vi "Set_OnlineData.vi"(8 "error in (no error)":errorcluster, 10 "Data_IN":T1={"Online"=TRUE, "Info"="", "OnlineData_State"=0} {"OnlineData_State" items=["Idle", "Manually", "Automatic"]}, 11 "MonSys_Server_Actor in":refnum<class "MonSys_Server_Actor.lvclass">) -> (0 "error out":errorcluster, 3 "MonSys_Server_Actor out":refnum<class "MonSys_Server_Actor.lvclass">)   [LabVIEW 2018, in "MonSys_Server_Actor.lvlib" / "MonSys_Server_Actor.lvclass"]
doc: "Replace SystemState DVR Data"
uses:
  MonSys_Server_Actor.lvclass
  _MonSys_LIB/OnlineData.ctl
  _MonSys_LIB/OnlineData_State.ctl
  MonSys_Server_Actor.lvclass/MonSys_Server_Actor.ctl
  _MonSys_LIB/_MonSys_LIB.lvlib
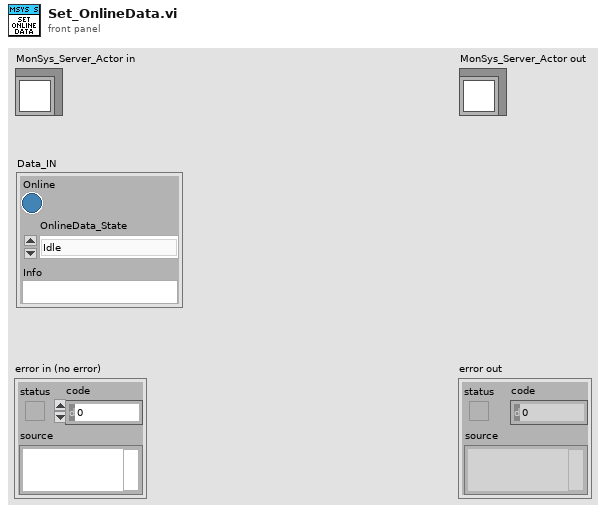
[diagram p1: front panel]
types:
  T1 = typedef "_MonSys_LIB.lvlib/OnlineData.ctl" = cluster{"Online":bool, "Info":string, "OnlineData_State":T2}
  T2 = typedef "_MonSys_LIB.lvlib/OnlineData_State.ctl" = u16
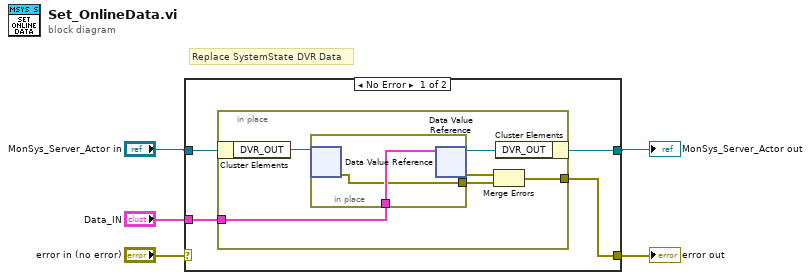
[diagram p0: block diagram]
diagram:
  # "Replace SystemState DVR Data"
  n1 = case shown="No Error" "error in (no error)" {
    selector: "error in (no error)" -> [_ w19]
    tunnel: [w7 w19] -> w3
    tunnel: [w6 w18] -> w2
    tunnel: "MonSys_Server_Actor in" -> [w9 w18]
    tunnel: "Data_IN" -> [w8 _]
    frame No Error {
      n2 = in-place {
        in-place-border: w8 -> [w14]
        in-place-border: [w11] -> w7
        n3 = in-place-cluster #1(w9) -> ("DVR_OUT"=w15:refnum<data-value>)
        n4 = in-place {
          in-place-border: w14 -> [w17]
          in-place-border: [w16] -> w13
          n5 = in-place-dvr #2(w15) -> (w16:errorcluster)  [unwired: 1 out]
          n6 = in-place-dvr #2(w17) -> (w10:refnum<data-value>, w12:errorcluster)
        }
        n7 = Merge Errors(w12, w13) -> (w11:errorcluster)
        n8 = in-place-cluster #1("DVR_OUT"=w10) -> (w6:refnum<class "MonSys_Server_Actor.lvclass">)
      }
    }
    frame Error {
    }
  }
  "error out" <- w3
  "MonSys_Server_Actor out" <- w2
